vi "4Pi Dual DM Control.vi"(7 "Calling VI Ref":refnum<vi>) -> ()   [LabVIEW 2016]
uses:
  4Pi Dual DM - Controls/4Pi Dual DM - Mirror Modes.ctl
  4Pi Dual DM - Controls/DM Max Voltages.ctl
  <vilib>/Utility/miscctls.llb/LVPointTypeDef.ctl
  4Pi Dual DM - Controls/4Pi Dual DM - Mirror Order.ctl
  4Pi Dual DM - Controls/4Pi Dual DM - Standard Action.ctl
  <vilib>/Analysis/baseanly.llb/Mean (DBL).vi
  <vilib>/Utility/file.llb/Read Delimited Spreadsheet (DBL).vi
  <vilib>/Utility/file.llb/Write Delimited Spreadsheet (DBL).vi
  <vilib>/Analysis/NI_AALBase.lvlib
panel:
  in  "DM Max Voltages (V)":T1
  in  "Scan Modes":bool
  in  "Astig On/Off":bool
  in  "Load Astig":bool
  in  "Active Mirror":enum32{"Mirror 1", "Mirror 2"}(radio)
  in  "Clear Modes":bool
  in  "Mirror Modes":T2
  in  "Load Modes":bool
  in  "Save Modes":bool
  in  "Load Flat":bool
  in  "Apply Zero":bool
  in  "Load V Map":bool
  in  "Save V Map":bool
  in  "Apply Flat":bool
  in  "Center Bias":bool
  in  "Quit":bool
  out "Pixel Map (-1 to 1)":dbl[][](graph)
  # "Mode"
  # "Amount (nm)"
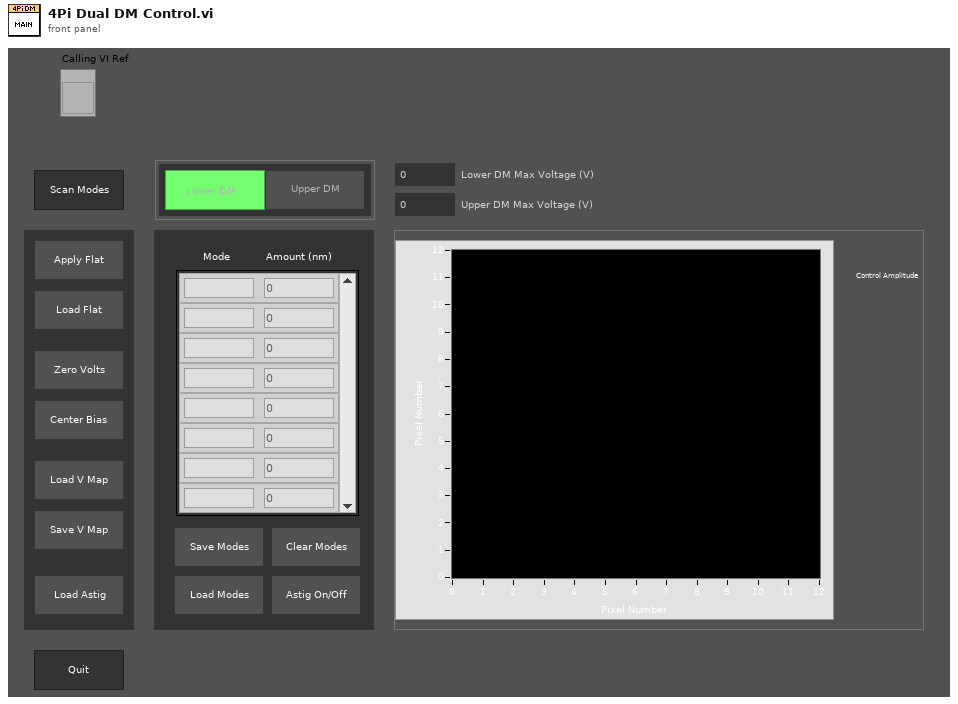
[diagram p1: front panel]
types:
  T1 = typedef "DM Max Voltages.ctl" = cluster{"Lower DM Max Voltage (V)":dbl, "Upper DM Max Voltage (V)":dbl}
  T2 = typedef "4Pi Dual DM - Mirror Modes.ctl" = cluster{"Mode":string, "Amplitude":dbl}[]
  T3 = typedef "4Pi Dual DM - Mirror Order.ctl" = cluster{"Flip Mirror Order":bool}
  T4 = enum16{"Always On", "Always Off", "Off While Running"}
  T5 = typedef "LVPointTypeDef.ctl" = cluster{"Horizontal":i16, "Vertical":i16}
  T6 = typedef "4Pi Dual DM - Standard Action.ctl" = enum16{"Read", "Write"}
  T7 = typedef "LVRectTypeDef.ctl" = cluster{"Left":i16, "Top":i16, "Right":i16, "Bottom":i16}
  T8 = typedef "LVBoundsTypeDef.ctl" = cluster{"Width":u32, "Height":u32}
  T9 = typedef "4Pi Dual DM - Mirror Modes DUAL.ctl" = cluster{"Mode":string, "Amplitude":dbl}[][]
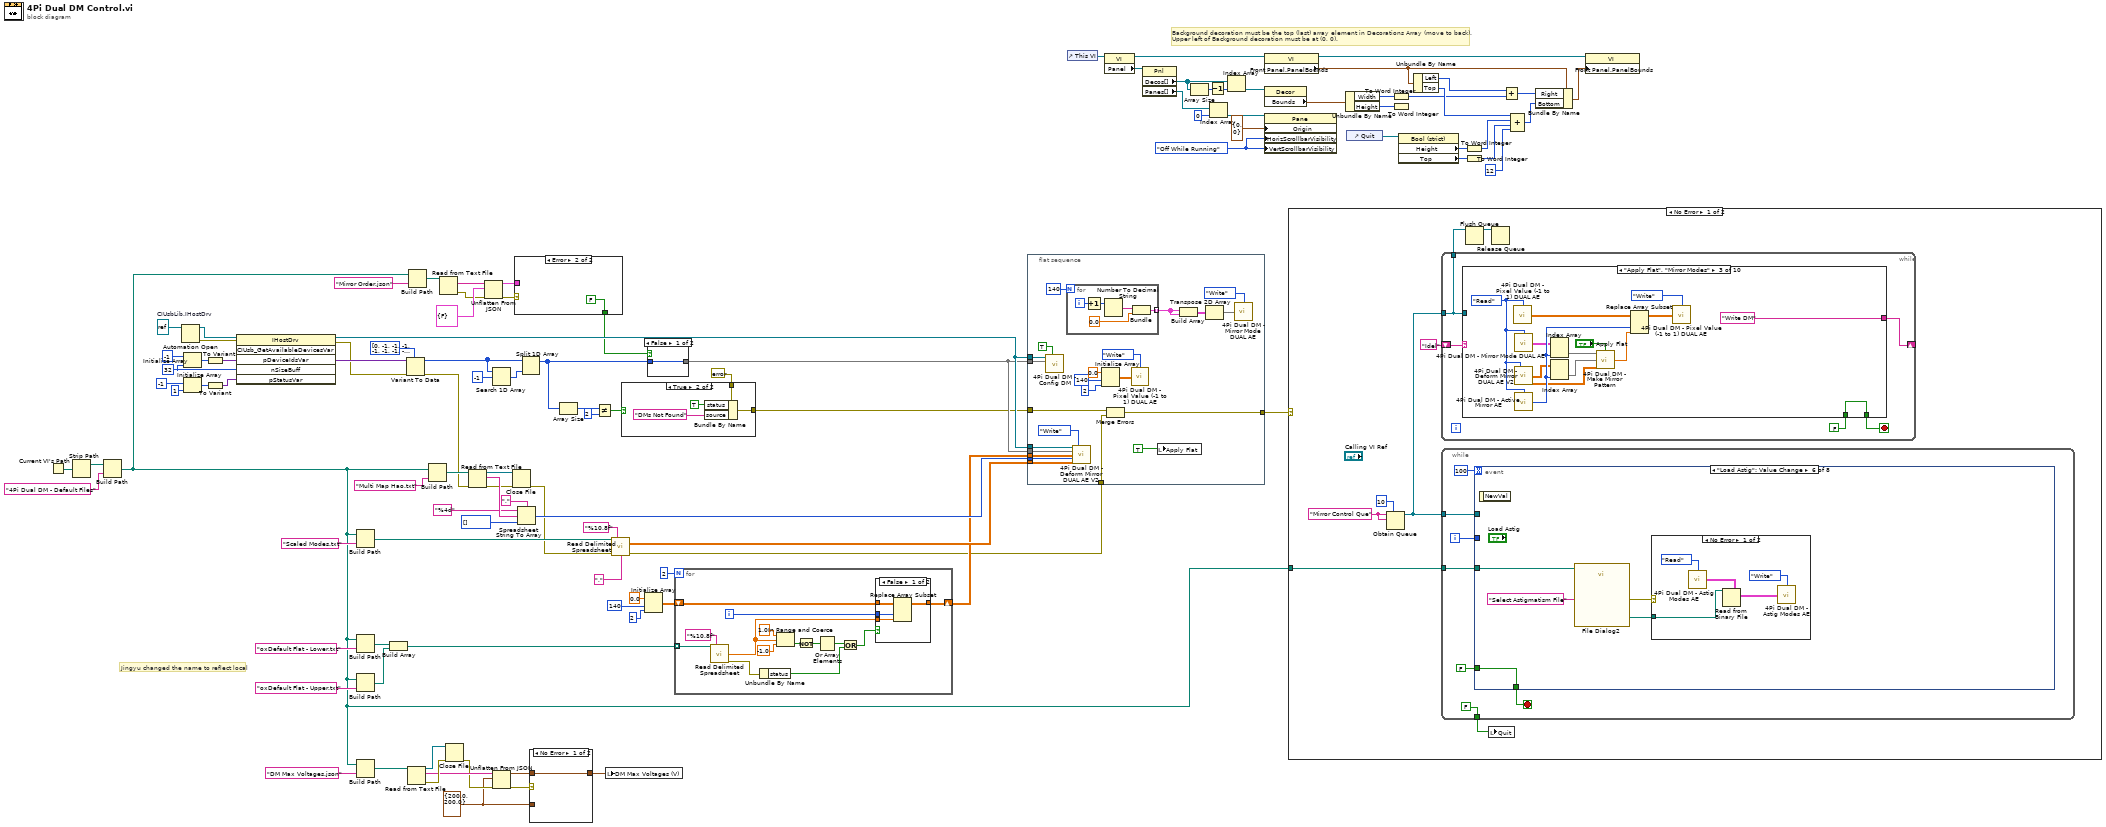
[diagram p0: block diagram]
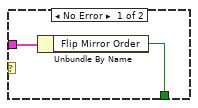
[diagram p2: hidden frame]
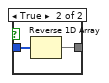
[diagram p4: hidden frame]
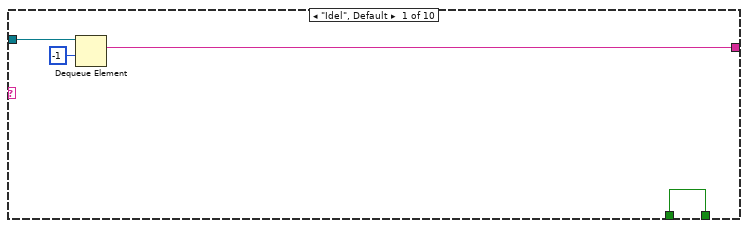
[diagram p5: hidden frame]
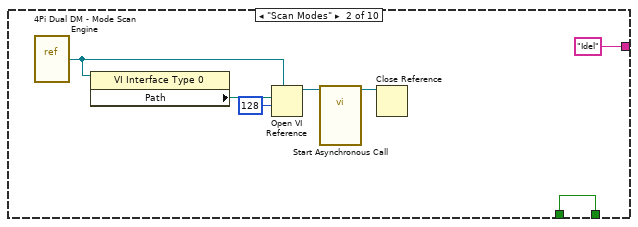
[diagram p6: hidden frame]
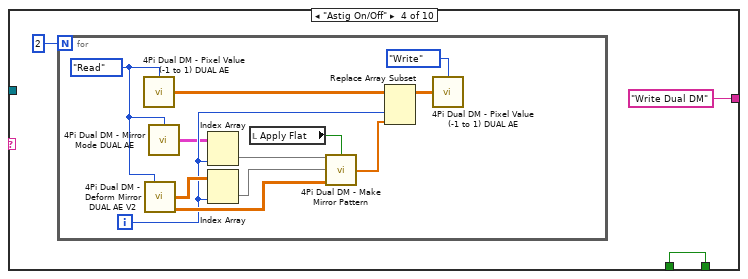
[diagram p7: hidden frame]
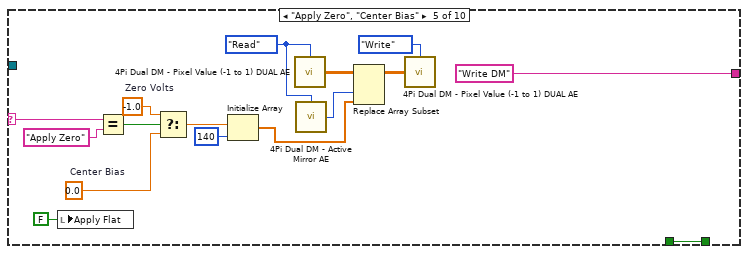
[diagram p8: hidden frame]
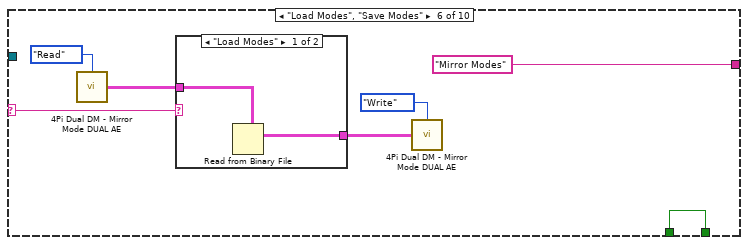
[diagram p9: hidden frame]
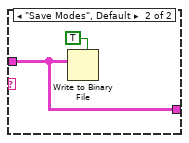
[diagram p10: hidden frame]
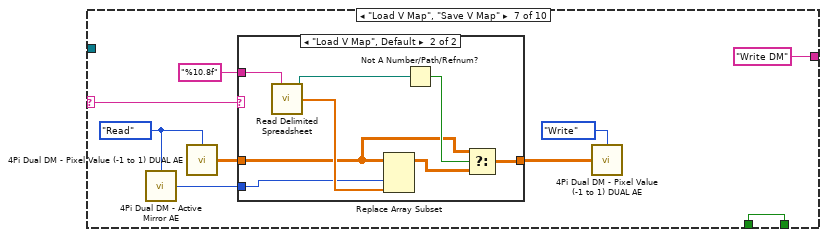
[diagram p11: hidden frame]
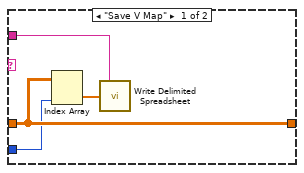
[diagram p12: hidden frame]
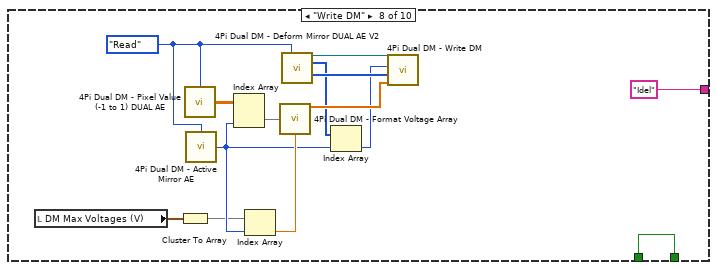
[diagram p13: hidden frame]
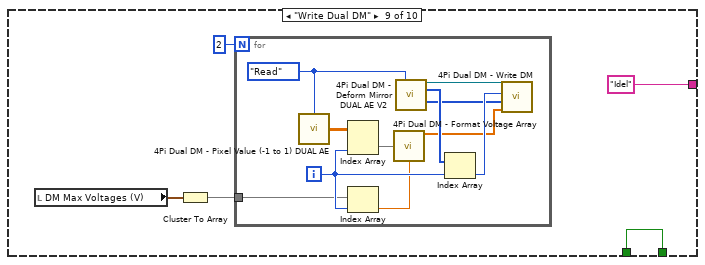
[diagram p14: hidden frame]
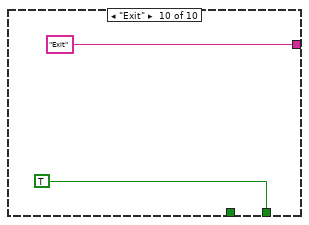
[diagram p15: hidden frame]
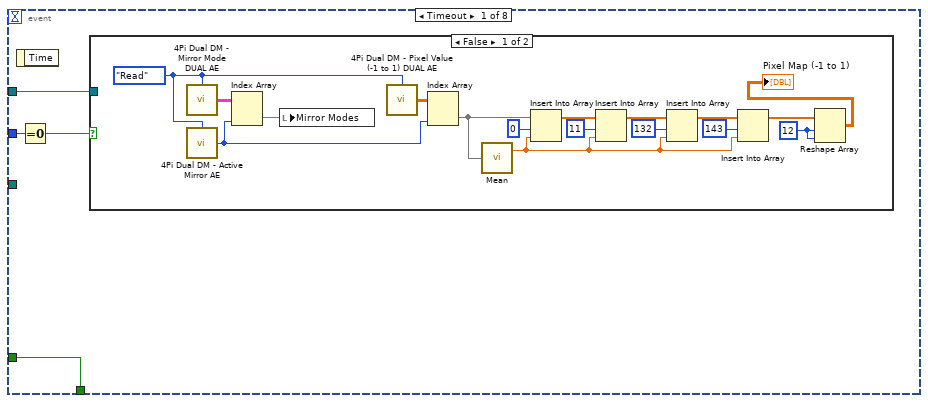
[diagram p16: hidden frame]
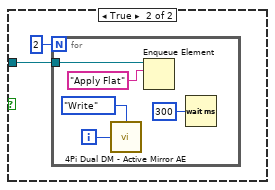
[diagram p17: hidden frame]
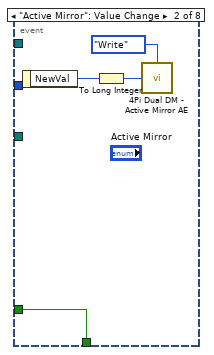
[diagram p18: hidden frame]
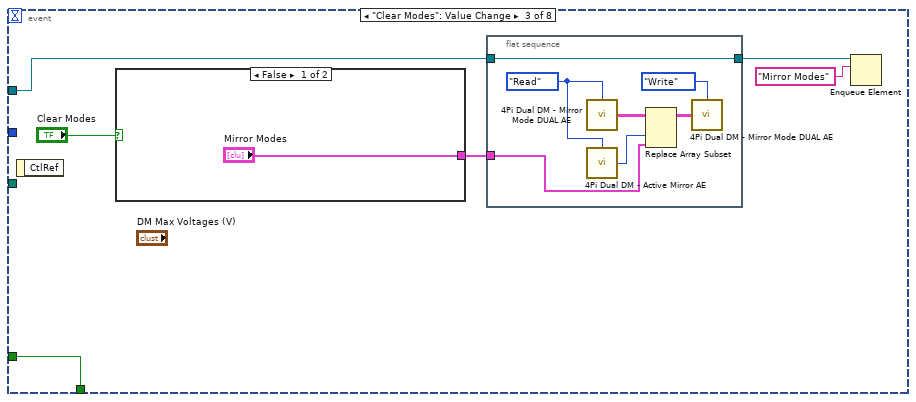
[diagram p19: hidden frame]
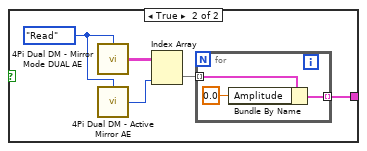
[diagram p20: hidden frame]
diagram:
  w6 = T1 {"Lower DM Max Voltage (V)"=200.0, "Upper DM Max Voltage (V)"=200.0} ("DM Max Voltages (V)")
  w71 = 32 ("dimension size")
  w62 = refnum<k7> refnum  # CIUsbLib.IHostDrv
  w88 = T4."Off While Running" ("Vertical Scrollbar Visibility")
  # "Jingyu changed the name to reflect local"
  # "Background decoration must be the top (last) array element in Decorations Array (move to back).\nUpper left of Background decoration must be at (0, 0)."
  n1 = Current VI's Path() -> (path=w46:path)
  n2 = Strip Path(path=w46) -> (stripped path=w47:path)  [unwired: 1 out]
  n3 = Build Path(base path=w47, name or relative path="4Pi Dual DM - Default Files") -> (appended path=w1:path)
  n4 = Automation Open(Automation Refnum=w62) -> (Automation Refnum=w67:refnum<k7>, error out=w68:errorcluster)  [unwired: 1 in, 2 out]
  n5 = Initialize Array(-1 ("element"), w71) -> (w64:i32[])
  n6 = Initialize Array(-1 ("element"), 1 ("dimension size")) -> (w63:i32[])
  n7 = To Variant(anything=w64) -> (Variant=w65:variant)
  n8 = To Variant(anything=w63) -> (Variant=w70:variant)
  n9 = invoke class="IHostDrv" method="CIUsb_GetAvailableDevicesVar"(reference=w67, error in=w68, "pDeviceIdsVar"=w65, "nSizeBuff"=w71, "pStatusVar"=w70) -> (reference out=w24:refnum<k7>, error out=w42:errorcluster, "pDeviceIdsVar"=w76:variant)  [unwired: 1 in, 3 out]
  n10 = Build Path(base path=w1, name or relative path="Scaled Modes.txt") -> (appended path=w53:path)
  n11 = Build Path(base path=w1, name or relative path="oxDefault Flat - Lower.txt") -> (appended path=w34:path)
  n12 = Build Path(base path=w1, name or relative path="oxDefault Flat - Upper.txt") -> (appended path=w33:path)
  n13 = Build Path(base path=w1, name or relative path="DM Max Voltages.json") -> (appended path=w12:path)
  n14 = Build Array(w34, w33) -> (w32:path[])
  n15 = Variant To Data(error in=w42, type=i32[] [0, -1, -1, -1, -1, -1, -1, -1, -1, -1, -1, -1, -1, -1, -1, -1, -1, -1, -1, -1, -1, -1, -1, -1, -1, -1, -1, -1, -1, -1, -1, -1] ("pDeviceIDs"), Variant=w76) -> (data=w74:i32[], error out=w30:errorcluster)
  n16 = Read from Text File(file (use dialog)=w12) -> (refnum out=w11:refnum<file>, text=w9:string, error out=w10:errorcluster)  [unwired: 3 in, 1 out]
  n17 = Build Path(base path=w1, name or relative path="Mirror Order.json") -> (appended path=w19:path)
  n18 = Build Path(base path=w1, name or relative path="Multi Map Hao.txt") -> (appended path=w55:path)
  n19 = Read from Text File(file (use dialog)=w19) -> (text=w18:string, error out=w14:errorcluster)  [unwired: 3 in, 2 out]
  n20 = Close File(refnum=w11, error in=w10) -> (error out=w8:errorcluster)  [unwired: 1 out]
  n21 = Read from Text File(file (use dialog)=w55, error in=w30) -> (refnum out=w57:refnum<file>, text=w61:string, error out=w56:errorcluster)  [unwired: 3 out]
  n22 = Unflatten From JSON(JSON string=w18, type and defaults=T3 {"Flip Mirror Order"=FALSE} ("Mirror Order"), error in (no error)=w14) -> (value=w16:T3, error out=w2:errorcluster)  [unwired: 4 in]
  n23 = Search 1D Array(1D array=w74, element=-1) -> (index of element=w73:i32)  [unwired: 1 in]
  n24 = Unflatten From JSON(JSON string=w9, type and defaults=w6, error in (no error)=w8) -> (value=w5:T1, error out=w7:errorcluster)  [unwired: 4 in]
  n25 = Close File(refnum=w57, error in=w56) -> (error out=w29:errorcluster)  [unwired: 1 out]
  n26 = case shown="Error" w2 {
    tunnel: w16 -> [w107 _]
    tunnel: [w106 FALSE ("Flip Mirror Order")] -> w15
    frame No Error {
      n27 = Unbundle By Name(w107) -> ("Flip Mirror Order"=w106:bool)
    }
    frame Error {
    }
  }
  n28 = Spreadsheet String To Array(delimiter (Tab)=",", format string="%4d", spreadsheet string=w61, array type (2D Dbl)=i32[] []) -> (array=w49:i32[])
  n29 = Split 1D Array(array=w74, index=w73) -> (first subarray=w48:i32[])  [unwired: 1 out]
  n30 = case shown="No Error" w7 {
    tunnel: w6 -> [_ w110]
    tunnel: w5 -> [w109 _]
    tunnel: [w109 w110] -> w4
    frame No Error {
    }
    frame Error {
    }
  }
  n31 = Array Size(array=w48) -> (size(s)=w28:i32)
  n32 = Not Equal?(x=w28, y=2) -> (x != y?=w26:bool)
  n33 = local write "DM Max Voltages (V)"(w4) -> ()
  n34 = call-poly <vilib>:"Read Delimited Spreadsheet.vi"("file path (dialog if empty)"=w53, "format (%.3f)"="%10.8f", "error in (no error)"=w29, "delimiter (\\t)"="," ("delimiter (\\t)")) -> ("all rows"=w51:dbl[][], "error out"=w22:errorcluster)  [unwired: 6 in, 4 out]
  n35 = case shown="True" w26 {
    tunnel: [w111 w113] -> w3
    tunnel: errorcluster {"status"=FALSE, "code"=0, "source"=""} ("error out") -> [w111 w112]
    frame False {
    }
    frame True {
      n36 = Bundle By Name(cluster=w112, "status"=TRUE, "source"="DMs Not Found" ("message")) -> (w113:errorcluster)
    }
  }
  n37 = Initialize Array(0.0 ("element"), 140 ("dimension size"), 2 ("dimension size")) -> (w37:dbl[][])
  n38 = case shown="False" w15 {
    tunnel: w48 -> [w116 w118]
    tunnel: [w116 w117] -> w21
    frame False {
    }
    frame True {
      n39 = Reverse 1D Array(array=w118) -> (reversed array=w117:i32[])
    }
  }
  n40 = for {
    N: 2 -> [_]
    shift-right: [w129] -> w31
    shift-left: w37 -> [w132]
    tunnel: w32 -> [w123] mode=indexing
    i -> [w131]
    n41 = call-poly <vilib>:"Read Delimited Spreadsheet.vi"("file path (dialog if empty)"=w123, "format (%.3f)"="%10.8f") -> ("first row"=w124:dbl[], "error out"=w122:errorcluster)  [unwired: 8 in, 4 out]
    n42 = Unbundle By Name(w122) -> ("status"=w120:bool)
    n43 = In Range and Coerce(upper limit=1.0, x=w124, lower limit=-1.0) -> (In Range?=w126:bool[])  [unwired: 1 out]
    n44 = Not(x=w126) -> (.not. x?=w127:bool[])
    n45 = Or Array Elements(Boolean array=w127) -> (logical OR=w121:bool)
    n46 = Or(x=w121, y=w120) -> (x .or. y?=w119:bool)
    n47 = case shown="False" w119 {
      tunnel: w132 -> [w136 w137]
      tunnel: w131 -> [w135 _]
      tunnel: [w134 w137] -> w129
      tunnel: w124 -> [w133 _]
      frame False {
        n48 = Replace Array Subset(array=w136, new element=w133, index (col)=w135) -> (w134:dbl[][])  [unwired: 1 in]
      }
      frame True {
      }
    }
  }
  n49 = flat-sequence {
    tunnel: w24 -> [w159]
    tunnel: w51 -> [w157]
    tunnel: w49 -> [w156]
    tunnel: w21 -> [w155]
    tunnel: w31 -> [w154]
    tunnel: w3 -> [w153]
    tunnel: w22 -> [w152]
    tunnel: w24 -> [w151]
    tunnel: [w145] -> w23
    tunnel: w21 -> [w144]
    frame #0 {
      n50 = call "4Pi Dual DM - Config DM.vi"("High Voltage"=TRUE, "Dev IDs"=w155, "Automation Refnum in"=w151) -> ()  [unwired: 7 in, 2 out]
      n51 = for {
        N: 140 -> [_]
        tunnel: [w161] -> w141 mode=indexing
        i -> [w165]
        n52 = Increment(x=w165) -> (x+1=w164:i32)
        n53 = Number To Decimal String(number=w164) -> (decimal integer string=w163:string)  [unwired: 1 in]
        n54 = Bundle(w163, 0.0) -> (w161:cluster{string, dbl})  [unwired: 1 in]
      }
      n55 = call "4Pi Dual DM - Deform Mirror DUAL AE V2.vi"("Refnum In"=w159, "Action"=4Pi_Dual_DM_-_Standard_Action."Write", "IDs In"=w144, "Flat Files In"=w154, "Multi Map Data In"=w156, "Mode Matrix"=w157) -> ()  [unwired: 5 in, 5 out]
      n56 = Initialize Array(0.0 ("element"), 140 ("dimension size"), 2 ("dimension size")) -> (w149:dbl[][])
      n57 = Merge Errors(w153, w152) -> (w145:errorcluster)
      n58 = call "4Pi Dual DM - Pixel Value (-1 to 1) DUAL AE.vi"("Action"=4Pi_Dual_DM_-_Standard_Action."Write", "Pixel Value (-1 to 1)"=w149) -> ()  [unwired: 13 in, 1 out]
      n59 = local write "Apply Flat"(TRUE ("Apply Flat")) -> ()
      n60 = Build Array(w141, w141) -> (w142:cluster{string, dbl}[][])
      n61 = Transpose 2D Array(2D array=w142) -> (transposed array=w143:cluster{string, dbl}[][])
      n62 = call "4Pi Dual DM - Mirror Mode DUAL AE.vi"("Action"=4Pi_Dual_DM_-_Standard_Action."Write", "Mirror Modes In"=w143) -> ()  [unwired: 13 in, 1 out]
    }
  }
  n63 = control-ref of="This VI"() -> (w80:refnum<vi>)
  n64 = property class="VI"(reference=w80) -> (reference out=w89:refnum<vi>, "Panel"=w81:refnum<vi>)  [unwired: 1 in, 1 out]
  n65 = property class="Pnl"(reference=w81) -> ("Decos[]"=w79:refnum<vi>[], "Panes[]"=w85:refnum<vi>[])  [unwired: 1 in, 2 out]
  n66 = Array Size(array=w79) -> (size(s)=w77:i32)
  n67 = Decrement(x=w77) -> (x-1=w78:i32)
  n68 = Index Array(array=w85, index=0) -> (element=w84:refnum<vi>)
  n69 = Index Array(array=w79, index=w78) -> (element=w87:refnum<vi>)
  n70 = property class="VI"(reference=w89) -> (reference out=w91:refnum<vi>, "Front Panel.PanelBounds"=w92:T7)  [unwired: 1 in, 1 out]
  n71 = property class="Decor"(reference=w87) -> ("Bounds"=w90:T8)  [unwired: 1 in, 2 out]
  n72 = property class="Pane"(reference=w84, "Origin"=T5 {"Horizontal"=0, "Vertical"=0}, "HorizScrollbarVisibility"=w88, "VertScrollbarVisibility"=w88) -> ()  [unwired: 1 in, 2 out]
  n73 = case shown="No Error" w23 {
    tunnel: w1 -> [w166 _]
    frame No Error {
      w173 = "Mirror Control Que" ("name (unnamed)")
      n74 = Obtain Queue(max queue size (-1, unlimited)=10, name (unnamed)=w173, element data type=w173) -> (queue out=w168:refnum<queue>)  [unwired: 2 in, 2 out]
      n75 = while {
        tunnel: w168 -> [w174]
        shift-right: [w178] -> _
        shift-left: "Idel" ("name (unnamed)") -> [w177]
        tunnel: [w174] -> w171
        stop <- w176 stop-if-true
        n76 = case shown="\"Apply Flat\", \"Mirror Modes\"" w177 {
          selector: w177 -> [_ _ _ _ w230 w237 w253 _ _ _]
          tunnel: w174 -> [w182 _ _ _ _ _ _ _ _ _]
          tunnel: [w180 "Idel" ("name (unnamed)") "Write DM" ("name (unnamed)") "Write Dual DM" ("name (unnamed)") "Write DM" ("name (unnamed)") "Mirror Modes" ("name (unnamed)") "Write DM" ("name (unnamed)") "Idel" ("name (unnamed)") "Idel" ("name (unnamed)") "Exit" ("name (unnamed)")] -> w178
          tunnel: [w179 w189 w202 w205 w234 w241 w254 w280 w285 TRUE] -> w176
          tunnel: FALSE -> [w179 w189 w202 w205 w234 w241 w254 w280 w285 _]
          frame "Idel", Default {
            n77 = Dequeue Element(queue=w182, timeout in ms (-1)=-1) -> (element=w180:string)  [unwired: 1 in, 3 out]
          }
          frame "Scan Modes" {
            n78 = vi-ref "4Pi Dual DM - Mode Scan Engine.vi"() -> (w183:refnum<vi>)
            n79 = property class="VI Interface Type 0"(reference=w183) -> ("Path"=w184:path)  [unwired: 1 in, 2 out]
            n80 = Open VI Reference(type specifier VI Refnum (for type only)=w183, vi path=w184, options=128) -> (vi reference=w186:refnum<vi>)  [unwired: 3 in, 1 out]
            n81 = call-by-ref "Start Asynchronous Call"(reference=w186) -> (reference out=w187:refnum<vi>)  [unwired: 17 in, 1 out]
            n82 = Close Reference(reference=w187) -> ()  [unwired: 1 in, 1 out]
          }
          frame "Apply Flat", "Mirror Modes" {
            w197 = 4Pi_Dual_DM_-_Standard_Action."Read" ("Action")
            n83 = call "4Pi Dual DM - Pixel Value (-1 to 1) DUAL AE.vi"("Action"=w197) -> ("Pixel Value (-1 to 1) Out"=w198:dbl[][])  [unwired: 14 in]
            n84 = call "4Pi Dual DM - Mirror Mode DUAL AE.vi"("Action"=w197) -> ("Mirror Modes Out"=w194:T9)  [unwired: 14 in]
            n85 = call "4Pi Dual DM - Deform Mirror DUAL AE V2.vi"("Action"=w197) -> ("Flat Files Out"=w192:dbl[][], "Mode Matrix Out"=w191:dbl[][])  [unwired: 10 in, 3 out]
            n86 = call "4Pi Dual DM - Active Mirror AE.vi"("Action"=w197) -> ("Active Mirror"=w200:i32)  [unwired: 14 in]
            n87 = Index Array(array=w194, index (col)=w200) -> (element=w195:cluster{"Mode":string, "Amplitude":dbl}[])  [unwired: 1 in]
            n88 = Index Array(array=w192, index (col)=w200) -> (element=w193:dbl[])  [unwired: 1 in]
            n89 = call "4Pi Dual DM - Make Mirror Pattern.vi"("Mirror Modes In"=w195, "Flat On?"="Apply Flat", "Flat File In"=w193, "Mirror Modes Array"=w191) -> ("Pixel Value U (-1 to 1)"=w199:dbl[])  [unwired: 11 in]
            n90 = Replace Array Subset(array=w198, new element=w199, index (col)=w200) -> (w201:dbl[][])  [unwired: 1 in]
            n91 = call "4Pi Dual DM - Pixel Value (-1 to 1) DUAL AE.vi"("Action"=4Pi_Dual_DM_-_Standard_Action."Write", "Pixel Value (-1 to 1)"=w201) -> ()  [unwired: 13 in, 1 out]
          }
          frame "Astig On/Off" {
            n92 = for {
              N: 2 -> [_]
              i -> [w209]
              w207 = 4Pi_Dual_DM_-_Standard_Action."Read" ("Action")
              n93 = call "4Pi Dual DM - Pixel Value (-1 to 1) DUAL AE.vi"("Action"=w207) -> ("Pixel Value (-1 to 1) Out"=w213:dbl[][])  [unwired: 14 in]
              n94 = call "4Pi Dual DM - Deform Mirror DUAL AE V2.vi"("Action"=w207) -> ("Flat Files Out"=w217:dbl[][], "Mode Matrix Out"=w218:dbl[][])  [unwired: 10 in, 3 out]
              n95 = call "4Pi Dual DM - Mirror Mode DUAL AE.vi"("Action"=w207) -> ("Mirror Modes Out"=w208:T9)  [unwired: 14 in]
              n96 = Index Array(array=w208, index (col)=w209) -> (element=w215:cluster{"Mode":string, "Amplitude":dbl}[])  [unwired: 1 in]
              n97 = Index Array(array=w217, index (col)=w209) -> (element=w216:dbl[])  [unwired: 1 in]
              n98 = local read "Apply Flat"() -> (w210:bool)
              n99 = call "4Pi Dual DM - Make Mirror Pattern.vi"("Mirror Modes In"=w215, "Flat On?"=w210, "Flat File In"=w216, "Mirror Modes Array"=w218) -> ("Pixel Value U (-1 to 1)"=w212:dbl[])  [unwired: 11 in]
              n100 = Replace Array Subset(array=w213, new element=w212, index (col)=w209) -> (w211:dbl[][])  [unwired: 1 in]
              n101 = call "4Pi Dual DM - Pixel Value (-1 to 1) DUAL AE.vi"("Action"=4Pi_Dual_DM_-_Standard_Action."Write", "Pixel Value (-1 to 1)"=w211) -> ()  [unwired: 13 in, 1 out]
            }
          }
          frame "Apply Zero", "Center Bias" {
            w222 = 4Pi_Dual_DM_-_Standard_Action."Read" ("Action")
            w226 = -1.0  # Zero Volts
            w228 = 0.0  # Center Bias
            n102 = local write "Apply Flat"(FALSE ("Apply Flat")) -> ()
            n103 = Equal?(x=w230, y="Apply Zero") -> (x = y?=w229:bool)
            n104 = Select(t=w226, s=w229, f=w228) -> (s? t:f=w227:dbl)
            n105 = Initialize Array(w227, 140 ("dimension size")) -> (w219:dbl[])
            n106 = call "4Pi Dual DM - Pixel Value (-1 to 1) DUAL AE.vi"("Action"=w222) -> ("Pixel Value (-1 to 1) Out"=w220:dbl[][])  [unwired: 14 in]
            n107 = call "4Pi Dual DM - Active Mirror AE.vi"("Action"=w222) -> ("Active Mirror"=w221:i32)  [unwired: 14 in]
            n108 = Replace Array Subset(array=w220, new element=w219, index (col)=w221) -> (w224:dbl[][])  [unwired: 1 in]
            n109 = call "4Pi Dual DM - Pixel Value (-1 to 1) DUAL AE.vi"("Action"=4Pi_Dual_DM_-_Standard_Action."Write", "Pixel Value (-1 to 1)"=w224) -> ()  [unwired: 13 in, 1 out]
          }
          frame "Load Modes", "Save Modes" {
            n110 = call "4Pi Dual DM - Mirror Mode DUAL AE.vi"("Action"=4Pi_Dual_DM_-_Standard_Action."Read") -> ("Mirror Modes Out"=w236:T9)  [unwired: 14 in]
            n111 = case shown="\"Load Modes\"" w237 {
              tunnel: w236 -> [w243 w244]
              tunnel: [w242 w244] -> w235
              frame "Load Modes" {
                n112 = Read from Binary File(5:w243) -> (2:w242:T9)  [unwired: 5 in, 3 out]
              }
              frame "Save Modes", Default {
                n113 = Write to Binary File(data=w244, 5:TRUE ("prepend array or string size? (T)")) -> ()  [unwired: 4 in, 3 out]
              }
            }
            n114 = call "4Pi Dual DM - Mirror Mode DUAL AE.vi"("Action"=4Pi_Dual_DM_-_Standard_Action."Write", "Mirror Modes In"=w235) -> ()  [unwired: 13 in, 1 out]
          }
          frame "Load V Map", "Save V Map" {
            w247 = 4Pi_Dual_DM_-_Standard_Action."Read" ("Action")
            n115 = call "4Pi Dual DM - Active Mirror AE.vi"("Action"=w247) -> ("Active Mirror"=w246:i32)  [unwired: 14 in]
            n116 = call "4Pi Dual DM - Pixel Value (-1 to 1) DUAL AE.vi"("Action"=w247) -> ("Pixel Value (-1 to 1) Out"=w251:dbl[][])  [unwired: 14 in]
            n117 = case shown="\"Load V Map\", Default" w253 {
              tunnel: w251 -> [w257 w259]
              tunnel: "%10.8f" -> [w258 w266]
              tunnel: [w257 w263] -> w248
              tunnel: w246 -> [w255 w260]
              frame "Save V Map" {
                n118 = Index Array(array=w257, index (col)=w255) -> (element=w256:dbl[])  [unwired: 1 in]
                n119 = call-poly <vilib>:"Write Delimited Spreadsheet.vi"("format (%.3f)"=w258, "1D data"=w256) -> ()  [unwired: 12 in, 2 out]
              }
              frame "Load V Map", Default {
                n120 = call-poly <vilib>:"Read Delimited Spreadsheet.vi"("format (%.3f)"=w266) -> ("new file path (Not A Path if cancelled)"=w265:path, "first row"=w261:dbl[])  [unwired: 9 in, 4 out]
                n121 = Replace Array Subset(array=w259, new element=w261, index (col)=w260) -> (w262:dbl[][])  [unwired: 1 in]
                n122 = Not A Number/Path/Refnum?(number/path/refnum=w265) -> (NaN/Path/Refnum?=w264:bool)
                n123 = Select(t=w259, s=w264, f=w262) -> (s? t:f=w263:dbl[][])
              }
            }
            n124 = call "4Pi Dual DM - Pixel Value (-1 to 1) DUAL AE.vi"("Action"=4Pi_Dual_DM_-_Standard_Action."Write", "Pixel Value (-1 to 1)"=w248) -> ()  [unwired: 13 in, 1 out]
          }
          frame "Write DM" {
            w273 = 4Pi_Dual_DM_-_Standard_Action."Read" ("Action")
            n125 = local read "DM Max Voltages (V)"() -> (w268:T1)
            n126 = Cluster To Array(cluster=w268) -> (array=w267:dbl[])
            n127 = call "4Pi Dual DM - Pixel Value (-1 to 1) DUAL AE.vi"("Action"=w273) -> ("Pixel Value (-1 to 1) Out"=w275:dbl[][])  [unwired: 14 in]
            n128 = call "4Pi Dual DM - Active Mirror AE.vi"("Action"=w273) -> ("Active Mirror"=w269:i32)  [unwired: 14 in]
            n129 = Index Array(array=w275, index (col)=w269) -> (element=w274:dbl[])  [unwired: 1 in]
            n130 = Index Array(array=w267, index=w269) -> (element=w270:dbl)
            n131 = call "4Pi Dual DM - Format Voltage Array.vi"("Pixel Level (-1 to 1)"=w274, "Max DM Voltage"=w270) -> ("Voltage Array (Volts)"=w276:dbl[])  [unwired: 12 in, 1 out]
            n132 = call "4Pi Dual DM - Deform Mirror DUAL AE V2.vi"("Action"=w273) -> ("Refnum Out"=w278:refnum<k7>, "IDs Out"=w272:i32[], "Multi Map Data Out"=w277:i32[])  [unwired: 10 in, 2 out]
            n133 = Index Array(array=w272, index=w269) -> (element=w271:i32)
            n134 = call "4Pi Dual DM - Write DM.vi"("reference in"=w278, "nDevId"=w271, "MultiDM  Mapping"=w277, "Voltage Array in"=w276) -> ()  [unwired: 2 in, 2 out]
          }
          frame "Write Dual DM" {
            n135 = local read "DM Max Voltages (V)"() -> (w282:T1)
            n136 = Cluster To Array(cluster=w282) -> (array=w281:dbl[])
            n137 = for {
              N: 2 -> [_]
              tunnel: w281 -> [w287]
              i -> [w288]
              w294 = 4Pi_Dual_DM_-_Standard_Action."Read" ("Action")
              n138 = call "4Pi Dual DM - Pixel Value (-1 to 1) DUAL AE.vi"("Action"=w294) -> ("Pixel Value (-1 to 1) Out"=w292:dbl[][])  [unwired: 14 in]
              n139 = Index Array(array=w292, index (col)=w288) -> (element=w293:dbl[])  [unwired: 1 in]
              n140 = Index Array(array=w287, index=w288) -> (element=w286:dbl)
              n141 = call "4Pi Dual DM - Format Voltage Array.vi"("Pixel Level (-1 to 1)"=w293, "Max DM Voltage"=w286) -> ("Voltage Array (Volts)"=w291:dbl[])  [unwired: 12 in, 1 out]
              n142 = call "4Pi Dual DM - Deform Mirror DUAL AE V2.vi"("Action"=w294) -> ("Refnum Out"=w289:refnum<k7>, "IDs Out"=w295:i32[], "Multi Map Data Out"=w290:i32[])  [unwired: 10 in, 2 out]
              n143 = Index Array(array=w295, index=w288) -> (element=w296:i32)
              n144 = call "4Pi Dual DM - Write DM.vi"("reference in"=w289, "nDevId"=w296, "MultiDM  Mapping"=w290, "Voltage Array in"=w291) -> ()  [unwired: 2 in, 2 out]
            }
          }
          frame "Exit" {
          }
        }
      }
      n145 = while {
        tunnel: w168 -> [w301]
        tunnel: [FALSE] -> w167
        tunnel: w166 -> [w299]
        i -> [w302]
        stop <- w305 stop-if-true
        n146 = event shown="[5] \"Load Astig\": Value Change" {
          selector: _ -> [_ _ _ _ _ _ _ _]
          dyn-events: _ -> [_ _ _ _ _ _ _ _]
          timeout: 100 -> [_ _ _ _ _ _ _ _]
          tunnel: [w309 w337 w343 w363 w368 w392 w401 w430] -> w305
          tunnel: FALSE -> [w309 w337 w343 w363 w368 w392 w401 _]
          tunnel: w302 -> [w308 _ _ _ _ _ _ _]
          tunnel: w301 -> [w306 _ w342 w362 _ _ w398 w428]
          tunnel: w299 -> [_ _ _ _ w367 w390 _ _]
          event Timeout {
            n147 = event-data() -> ()  [unwired: 1 in, 1 out]
            n148 = Equal To 0?(x=w308) -> (x = 0?=w307:bool)
            n149 = case shown="False" w307 {
              tunnel: w306 -> [_ w328]
              frame False {
                w322 = 12 ("dimension size")
                w323 = 4Pi_Dual_DM_-_Standard_Action."Read" ("Action")
                n150 = call "4Pi Dual DM - Mirror Mode DUAL AE.vi"("Action"=w323) -> ("Mirror Modes Out"=w310:T9)  [unwired: 14 in]
                n151 = call "4Pi Dual DM - Active Mirror AE.vi"("Action"=w323) -> ("Active Mirror"=w325:i32)  [unwired: 14 in]
                n152 = Index Array(array=w310, index (col)=w325) -> (element=w311:cluster{"Mode":string, "Amplitude":dbl}[])  [unwired: 1 in]
                n153 = local write "Mirror Modes"(w311) -> ()
                n154 = call "4Pi Dual DM - Pixel Value (-1 to 1) DUAL AE.vi"("Action"=w323) -> ("Pixel Value (-1 to 1) Out"=w324:dbl[][])  [unwired: 14 in]
                n155 = Index Array(array=w324, index (col)=w325) -> (element=w326:dbl[])  [unwired: 1 in]
                n156 = call-poly <vilib>:"Mean.vi"("X"=w326) -> ("mean"=w320:dbl)  [unwired: 1 out]
                n157 = Insert Into Array(array=w326, index=0, new element=w320) -> (w315:dbl[])
                n158 = Insert Into Array(array=w315, index=11, new element=w320) -> (w317:dbl[])
                n159 = Insert Into Array(array=w317, index=132, new element=w320) -> (w319:dbl[])
                n160 = Insert Into Array(array=w319, index=143, new element=w320) -> (w312:dbl[])
                n161 = Reshape Array(w312, w322, w322) -> (→"Pixel Map (-1 to 1)":dbl[][])
              }
              frame True {
                n162 = for {
                  N: 2 -> [_]
                  tunnel: w328 -> [w333]
                  i -> [w329]
                  n163 = call "4Pi Dual DM - Active Mirror AE.vi"("Action"=4Pi_Dual_DM_-_Standard_Action."Write", "Active Mirror In"=w329) -> ()  [unwired: 13 in, 1 out]
                  n164 = Enqueue Element(queue=w333, element="Apply Flat") -> ()  [unwired: 2 in, 3 out]
                  n165 = Wait (ms)(milliseconds to wait=u32 300) -> ()  [unwired: 1 out]
                }
              }
            }
          }
          event "Active Mirror": Value Change {
            n166 = event-data() -> ("NewVal"=w336:enum32{"Mirror 1", "Mirror 2"})  [unwired: 1 in]
            n167 = To Long Integer(number=w336) -> (32bit integer=w335:i32)
            n168 = call "4Pi Dual DM - Active Mirror AE.vi"("Action"=4Pi_Dual_DM_-_Standard_Action."Write", "Active Mirror In"=w335) -> ()  [unwired: 13 in, 1 out]
          }
          event "Clear Modes": Value Change {
            n169 = event-data() -> ()  [unwired: 1 in, 1 out]
            n170 = case shown="False" "Clear Modes" {
              tunnel: ["Mirror Modes" w345] -> w338
              frame False {
              }
              frame True {
                w348 = 4Pi_Dual_DM_-_Standard_Action."Read" ("Action")
                n171 = call "4Pi Dual DM - Mirror Mode DUAL AE.vi"("Action"=w348) -> ("Mirror Modes Out"=w347:T9)  [unwired: 14 in]
                n172 = call "4Pi Dual DM - Active Mirror AE.vi"("Action"=w348) -> ("Active Mirror"=w349:i32)  [unwired: 14 in]
                n173 = Index Array(array=w347, index (col)=w349) -> (element=w346:cluster{"Mode":string, "Amplitude":dbl}[])  [unwired: 1 in]
                n174 = for {
                  tunnel: w346 -> [w352] mode=indexing
                  tunnel: [w350] -> w345 mode=indexing
                  n175 = Bundle By Name(cluster=w352, "Amplitude"=0.0) -> (w350:cluster{"Mode":string, "Amplitude":dbl})
                }
              }
            }
            n176 = flat-sequence {
              tunnel: w338 -> [w353]
              tunnel: w342 -> [w359]
              tunnel: [w359] -> w340
              frame #0 {
                w356 = 4Pi_Dual_DM_-_Standard_Action."Read" ("Action")
                n177 = call "4Pi Dual DM - Mirror Mode DUAL AE.vi"("Action"=w356) -> ("Mirror Modes Out"=w355:T9)  [unwired: 14 in]
                n178 = call "4Pi Dual DM - Active Mirror AE.vi"("Action"=w356) -> ("Active Mirror"=w357:i32)  [unwired: 14 in]
                n179 = Replace Array Subset(array=w355, new element=w353, index (col)=w357) -> (w358:T9)  [unwired: 1 in]
                n180 = call "4Pi Dual DM - Mirror Mode DUAL AE.vi"("Action"=4Pi_Dual_DM_-_Standard_Action."Write", "Mirror Modes In"=w358) -> ()  [unwired: 13 in, 1 out]
              }
            }
            n181 = Enqueue Element(queue=w340, element="Mirror Modes") -> ()  [unwired: 2 in, 3 out]
          }
          event "Apply Flat", "Center Bias", "Apply Zero", "Save V Map", "Save Modes", "Load Modes", "Load V Map", "Scan Modes": Value Change {
            n182 = event-data() -> ("CtlRef"=w361:refnum<vi>)  [unwired: 1 in]
            n183 = property class="Bool"(reference=w361) -> ("Label.Text"=w360:string)  [unwired: 1 in, 2 out]
            n184 = Enqueue Element(queue=w362, element=w360) -> ()  [unwired: 2 in, 3 out]
          }
          event "Load Flat": Value Change {
            n185 = event-data() -> ()  [unwired: 1 in, 1 out]
            n186 = call "File Dialog"("start path"=w367, "prompt"="Select Flat File") -> ("selected path"=w364:path, "error out"=w365:errorcluster)  [unwired: 10 in, 2 out]
            n187 = case shown="No Error" w365 {
              tunnel: w364 -> [w369 _]
              frame No Error {
                w376 = 4Pi_Dual_DM_-_Standard_Action."Read" ("Action")
                n188 = call-poly <vilib>:"Read Delimited Spreadsheet.vi"("file path (dialog if empty)"=w369, "format (%.3f)"="%10.8f") -> ("first row"=w385:dbl[])  [unwired: 8 in, 5 out]
                n189 = In Range and Coerce(upper limit=1.0, x=w385, lower limit=-1.0) -> (coerced(x)=w370:dbl[], In Range?=w382:bool[])
                n190 = call "4Pi Dual DM - Deform Mirror DUAL AE V2.vi"("Action"=w376) -> ("Refnum Out"=w371:refnum<k7>, "IDs Out"=w372:i32[], "Flat Files Out"=w377:dbl[][], "Multi Map Data Out"=w373:i32[], "Mode Matrix Out"=w374:dbl[][])  [unwired: 10 in]
                n191 = call "4Pi Dual DM - Active Mirror AE.vi"("Action"=w376) -> ("Active Mirror"=w379:i32)  [unwired: 14 in]
                n192 = Not(x=w382) -> (.not. x?=w381:bool[])
                n193 = Replace Array Subset(array=w377, new element=w370, index (col)=w379) -> (w378:dbl[][])  [unwired: 1 in]
                n194 = Or Array Elements(Boolean array=w381) -> (logical OR=w380:bool)
                n195 = call "4Pi Dual DM - Deform Mirror DUAL AE V2.vi"("Refnum In"=w371, "Action"=4Pi_Dual_DM_-_Standard_Action."Write", "IDs In"=w372, "Flat Files In"=w378, "Multi Map Data In"=w373, "Mode Matrix"=w374) -> ()  [unwired: 5 in, 5 out]
                n196 = case shown="True" w380 {
                  frame False {
                  }
                  frame True {
                    n197 = One Button Dialog(message="Flat File Out of Range [-1, 1]") -> ()  [unwired: 1 in, 1 out]
                  }
                }
              }
              frame Error {
              }
            }
          }
          event "Load Astig": Value Change {
            n198 = event-data() -> ()  [unwired: 1 in, 1 out]
            n199 = call "File Dialog2"("start path"=w390, "prompt"="Select Astigmatism File") -> ("selected path"=w388:path, "error out"=w389:errorcluster)  [unwired: 10 in, 2 out]
            n200 = case shown="No Error" w389 {
              tunnel: w388 -> [w393 _]
              frame No Error {
                n201 = call "4Pi Dual DM - Astig Modes AE.vi"("Action"=4Pi_Dual_DM_-_Standard_Action."Read") -> ("Mirror Modes Out"=w397:T9)  [unwired: 14 in]
                n202 = Read from Binary File(5:w397, 11:w393) -> (2:w394:T9)  [unwired: 4 in, 3 out]
                n203 = call "4Pi Dual DM - Astig Modes AE.vi"("Action"=4Pi_Dual_DM_-_Standard_Action."Write", "Mirror Modes In"=w394) -> ()  [unwired: 13 in, 1 out]
              }
              frame Error {
              }
            }
          }
          event "Astig On/Off": Value Change {
            n204 = event-data() -> ()  [unwired: 1 in, 1 out]
            n205 = case shown="True" "Astig On/Off" {
              tunnel: [w406 w418] -> w399
              frame False {
                n206 = for {
                  N: 2 -> [_]
                  tunnel: [w409] -> w407 mode=indexing
                  i -> [w410]
                  n207 = call "4Pi Dual DM - Mirror Mode DUAL AE.vi"("Action"=4Pi_Dual_DM_-_Standard_Action."Read") -> ("Mirror Modes Out"=w412:T9)  [unwired: 14 in]
                  n208 = Index Array(array=w412, index (col)=w410) -> (element=w413:cluster{"Mode":string, "Amplitude":dbl}[])  [unwired: 1 in]
                  n209 = for {
                    tunnel: w413 -> [w416] mode=indexing
                    tunnel: [w414] -> w409 mode=indexing
                    n210 = Bundle By Name(cluster=w416, "Amplitude"=0.0) -> (w414:cluster{"Mode":string, "Amplitude":dbl})
                  }
                }
                n211 = Transpose 2D Array(2D array=w407) -> (transposed array=w406:cluster{"Mode":string, "Amplitude":dbl}[][])
              }
              frame True {
                n212 = call "4Pi Dual DM - Astig Modes AE.vi"("Action"=4Pi_Dual_DM_-_Standard_Action."Read") -> ("Mirror Modes Out"=w418:T9)  [unwired: 14 in]
              }
            }
            n213 = flat-sequence {
              tunnel: w399 -> [w403]
              tunnel: w398 -> [w404]
              frame #0 {
                n214 = call "4Pi Dual DM - Mirror Mode DUAL AE.vi"("Action"=4Pi_Dual_DM_-_Standard_Action."Write", "Mirror Modes In"=w403) -> ()  [unwired: 13 in, 1 out]
              }
              frame #1 {
                n215 = Enqueue Element(queue=w404, element="Astig On/Off") -> ()  [unwired: 2 in, 3 out]
              }
            }
          }
          event "Quit": Value Change {
            n216 = event-data() -> ("NewVal"=w430:bool)  [unwired: 1 in]
            n217 = for {
              N: 2 -> [_]
              tunnel: w428 -> [w436]
              tunnel: [w431] -> w419
              i -> [w432]
              n218 = call "4Pi Dual DM - Active Mirror AE.vi"("Action"=4Pi_Dual_DM_-_Standard_Action."Write", "Active Mirror In"=w432) -> ()  [unwired: 13 in, 1 out]
              n219 = Enqueue Element(queue=w436, element="Apply Zero") -> (queue out=w431:refnum<queue>)  [unwired: 2 in, 2 out]
              n220 = Wait (ms)(milliseconds to wait=u32 300) -> ()  [unwired: 1 out]
            }
            n221 = Enqueue Element(queue=w419, element="Exit") -> (error out=w423:errorcluster)  [unwired: 2 in, 2 out]
            n222 = call "4Pi Dual DM - Deform Mirror DUAL AE V2.vi"("Action"=4Pi_Dual_DM_-_Standard_Action."Read") -> ("Refnum Out"=w426:refnum<k7>, "IDs Out"=w421:i32[])  [unwired: 10 in, 3 out]
            n223 = call "4Pi Dual DM - Config DM.vi"("High Voltage"=FALSE, "error in (no error)"=w423, "Dev IDs"=w421, "Automation Refnum in"=w426) -> ("error out"=w422:errorcluster, "Automation Refnum out"=w425:refnum<k7>)  [unwired: 6 in]
            n224 = Close Reference(reference=w425, error in (no error)=w422) -> ()  [unwired: 1 out]
          }
        }
      }
      n225 = Flush Queue(queue=w171) -> (queue out=w170:refnum<queue>)  [unwired: 1 in, 2 out]
      n226 = local write "Quit"(w167) -> ()
      n227 = Release Queue(queue=w170) -> ()  [unwired: 2 in, 3 out]
    }
    frame Error {
      n228 = One Button Dialog(message="DMs not found.") -> ()  [unwired: 1 in, 1 out]
    }
  }
  n229 = Unbundle By Name(w90) -> ("Width"=w95:u32, "Height"=w98:u32)
  n230 = control-ref of="Quit"() -> (w82:refnum<vi>)
  n231 = To Word Integer(number=w95) -> (16bit integer=w97:i16)
  n232 = To Word Integer(number=w98) -> ()  [unwired: 1 out]
  n233 = property class="Bool (strict)"(reference=w82) -> ("Height"=w100:u32, "Top"=w101:i32)  [unwired: 1 in, 2 out]
  n234 = Unbundle By Name(w92) -> ("Left"=w94:i16, "Top"=w105:i16)
  n235 = To Word Integer(number=w100) -> (16bit integer=w103:i16)
  n236 = To Word Integer(number=w101) -> (16bit integer=w104:i16)
  n237 = Add(x=w94, y=w97) -> (x+y=w96:i16)
  n238 = Compound Arithmetic op=ADD(w105, w103, w104, i16 12 ("y")) -> (w99:i16)
  n239 = Bundle By Name(cluster=w92, "Right"=w96, "Bottom"=w99) -> (w93:T7)
  n240 = property class="VI"(reference=w91, "Front Panel.PanelBounds"=w93) -> ()  [unwired: 1 in, 2 out]
